vi "uni1 (SubVI).vi"(0 "start":cluster{"x":dbl, "y":dbl}, 6 "xmax":dbl=1.0, 9 "xmin":dbl, 10 "dencity":i32=128, 11 "goal":cluster{"x":dbl, "y":dbl}) -> (3 "Array":cluster{"x":dbl, "y":dbl}[](array[cluster]))   [LabVIEW 2011]
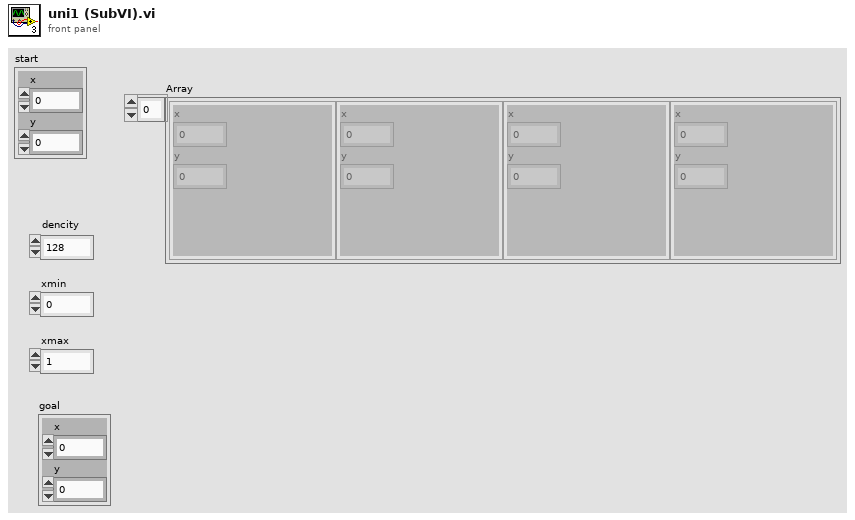
[diagram p1: front panel]
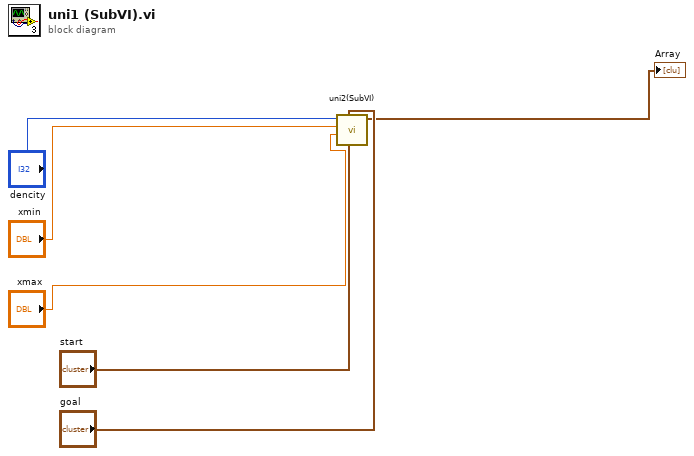
[diagram p0: block diagram]
diagram:
  n1 = call "uni2(SubVI).vi"("start"="start", "goal"="goal", "xmax"="xmax", "xmin"="xmin", "dencity"="dencity") -> ("Array"=→"Array":cluster{"x":dbl, "y":dbl}[])  [unwired: 6 in]
